vi "New Terminals Updated.vi"(7 "Prev Terminal Count":i32, 8 "error in (no error)":errorcluster, 9 "Analytics Button Pressed?":bool, 10 "Samples to display":i32, 11 "Terminal Count":u32) -> (0 "error out":errorcluster, 1 "Top/Bottom":bool, 2 "Values Inserted":u32, 3 "No Of New Terminals":u32, 5 "Prev Terminal Count":u32)   [LabVIEW 2019, in "Zen Analytics.lvlib" / "Zen Analytics.lvclass"]
uses:
  Zen Analytics.lvclass
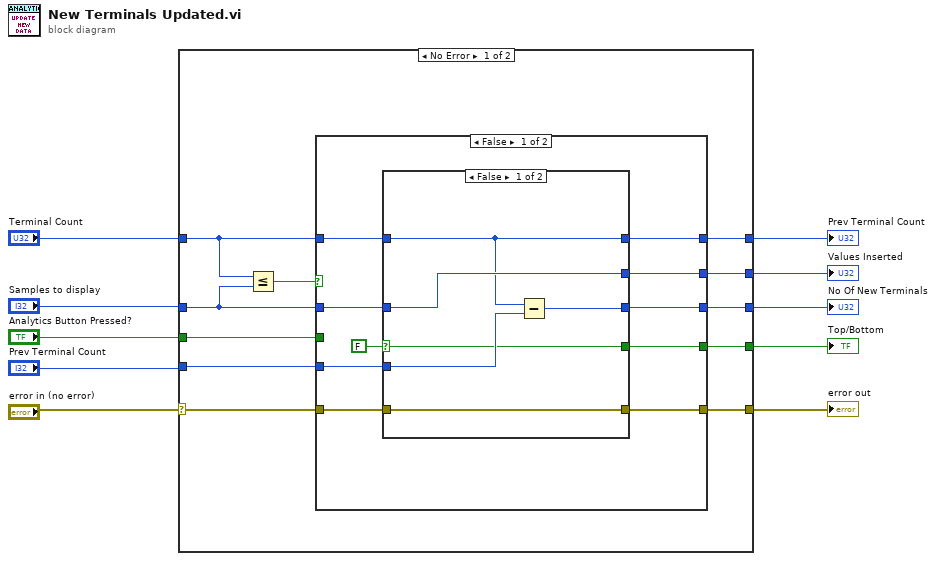
[diagram p0: block diagram]
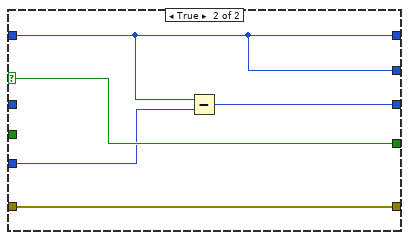
[diagram p3: hidden frame]
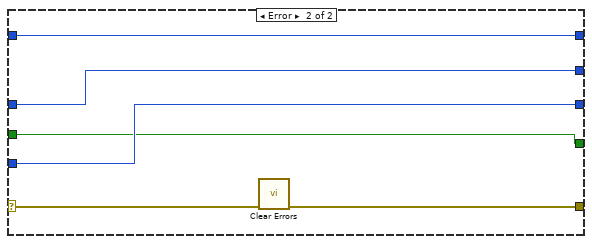
[diagram p4: hidden frame]
diagram:
  n1 = case shown="No Error" "error in (no error)" {
    selector: "error in (no error)" -> [w21 w52]
    tunnel: [w20 w47] -> w1
    tunnel: "Analytics Button Pressed?" -> [w19 w50]
    tunnel: [w18 w51] -> w3
    tunnel: "Prev Terminal Count" -> [w17 w51]
    tunnel: [w16 w49] -> w5
    tunnel: "Terminal Count" -> [w13 w49]
    tunnel: "Samples to display" -> [w12 w48]
    tunnel: [w15 w50] -> w2
    tunnel: [w11 w48] -> w4
    frame No Error {
      n2 = Less Or Equal?(x=w13, y=w12) -> (x <= y?=w14:bool)
      n3 = case shown="False" w14 {
        selector: w14 -> [_ w45]
        tunnel: w21 -> [w31 w46]
        tunnel: [w30 w46] -> w20
        tunnel: w19 -> [_ _]
        tunnel: [w29 w43] -> w18
        tunnel: w17 -> [w28 w44]
        tunnel: [w27 w42] -> w16
        tunnel: w13 -> [w23 w42]
        tunnel: w12 -> [w26 _]
        tunnel: [w25 w45] -> w15
        tunnel: [w24 w42] -> w11
        frame False {
          n4 = case shown="False" FALSE {
            selector: FALSE -> [w34 w38]
            tunnel: w31 -> [w35 w41]
            tunnel: [w35 w41] -> w30
            tunnel: [w36 w40] -> w29
            tunnel: [w32 w39] -> w27
            tunnel: w28 -> [w37 _]
            tunnel: w26 -> [w33 w40]
            tunnel: [w34 w38] -> w25
            tunnel: [w33 w40] -> w24
            tunnel: w23 -> [w32 w39]
            frame False {
              n5 = Subtract(x=w32, y=w37) -> (x-y=w36:u32)
            }
            frame True {
            }
          }
        }
        frame True {
          n6 = Subtract(x=w42, y=w44) -> (x-y=w43:u32)
        }
      }
    }
    frame Error {
      n7 = call <vilib>:"Clear Errors.vi"("error in (no error)"=w52) -> ("error out"=w47:errorcluster)  [unwired: 5 in, 1 out]
    }
  }
  "No Of New Terminals" <- w3
  "error out" <- w1
  "Prev Terminal Count" <- w5
  "Top/Bottom" <- w2
  "Values Inserted" <- w4
